vi "TrajAverage.vi"(8 "error in (no error)":errorcluster, 11 "ForceField in":refnum<class "ForceField.lvclass">) -> (0 "error out":errorcluster, 3 "ForceField out":refnum<class "ForceField.lvclass">)   [LabVIEW 2014, in "ForceField.lvclass"]
uses:
  ForceField.lvclass
  TypeDef/AnkleTrajPt.ctl
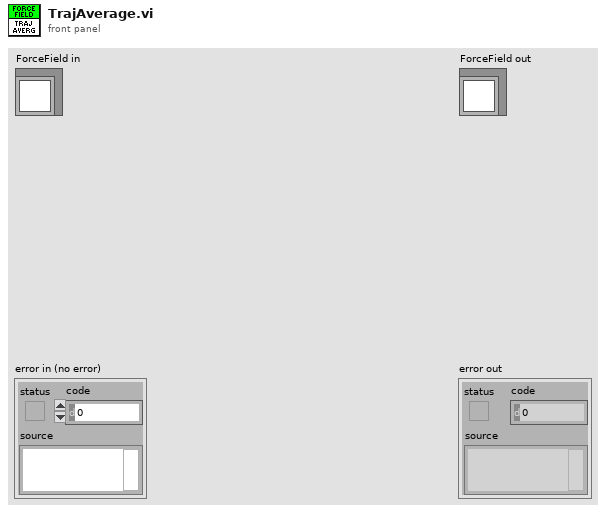
[diagram p1: front panel]
types:
  T1 = typedef "ForceField.lvclass/AnkleTrajPt.ctl" = cluster{"P1":dbl[], "P2":dbl[], "P1-P2":dbl[], "(P1-P2)^2":dbl}
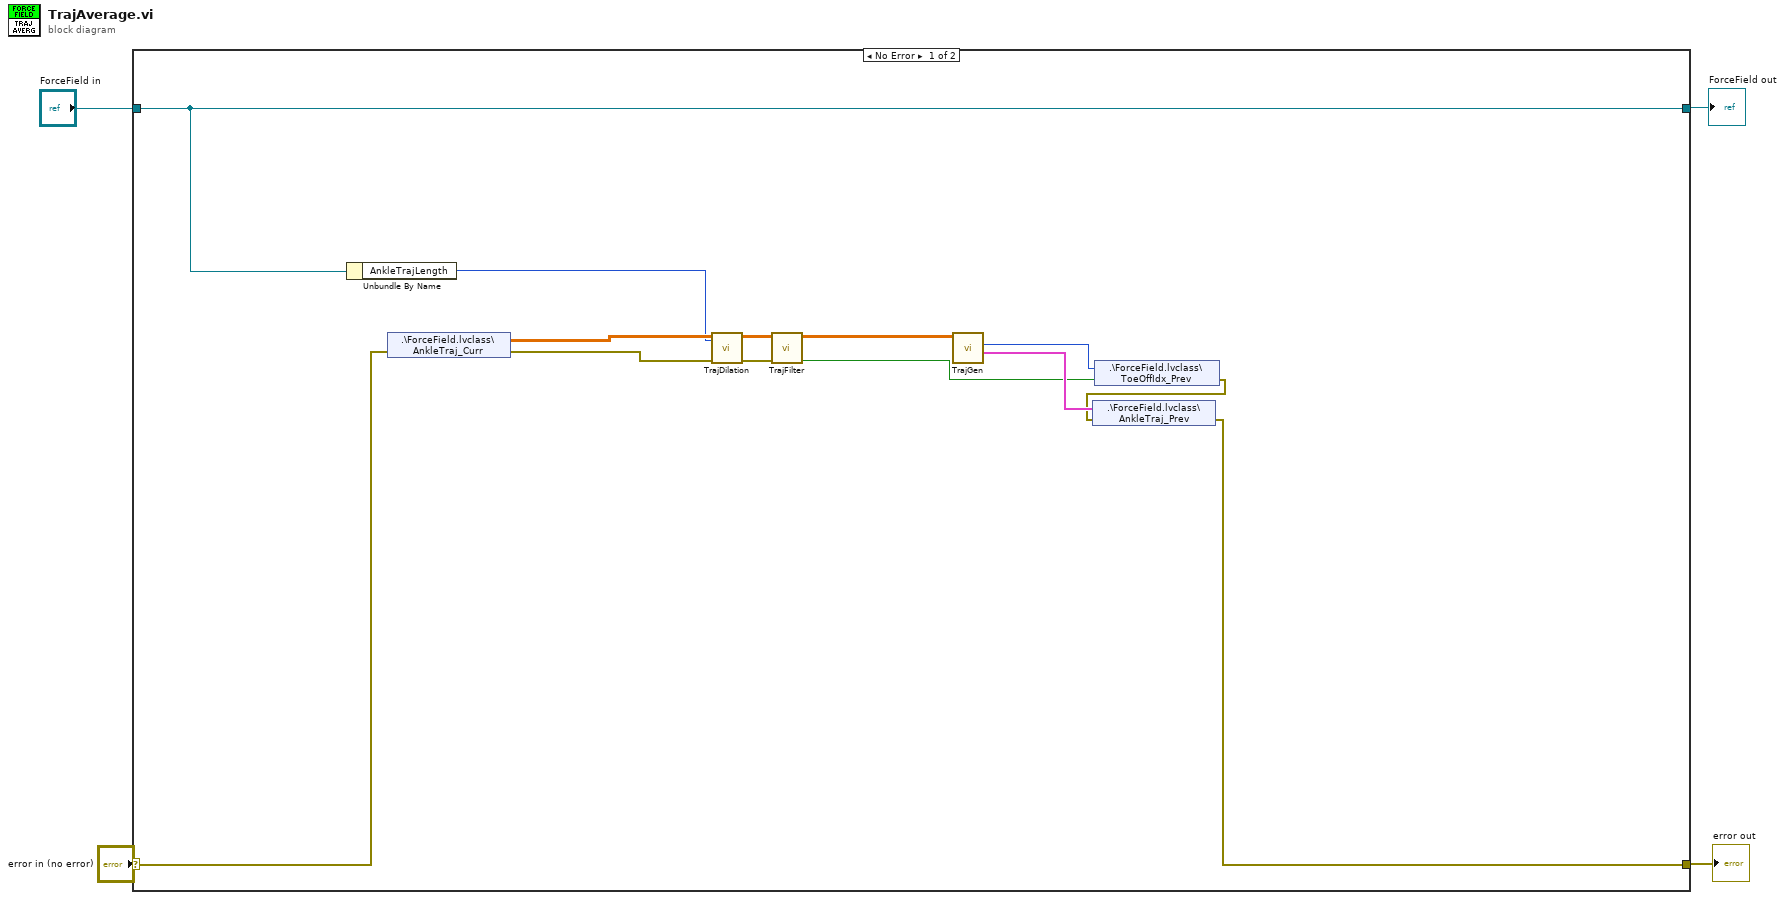
[diagram p0: block diagram]
diagram:
  n1 = case shown="No Error" "error in (no error)" {
    selector: "error in (no error)" -> [w14 w18]
    tunnel: [w7 w18] -> w3
    tunnel: [w13 w17] -> w1
    tunnel: "ForceField in" -> [w13 w17]
    frame No Error {
      n2 = Unbundle By Name(w13) -> ("AnkleTrajLength"=w12:i32)
      n3 = shared-variable ".\\ForceField.lvclass\\AnkleTraj_Curr"(error in=w14) -> (w16:dbl[][], error out=w6:errorcluster)
      n4 = call "TrajDilation.vi"("Length"=w12, "TrajBeforeDilation"=w16) -> ("TrajAfterDilation"=w15:dbl[][])  [unwired: 9 in]
      n5 = call "TrajFilter.vi"("AnkleTraj_Init"=w6, "CurrentTraj"=w15) -> ("AnkleTraj_Init 2"=w5:bool, "AverageTraj"=w11:dbl[][])  [unwired: 6 in]
      n6 = call "TrajGen.vi"("AnkleTraj"=w11) -> ("AnkleTraj"=w10:T1[], "ToeOffIdx"=w9:i32)  [unwired: 5 in, 2 out]
      n7 = shared-variable ".\\ForceField.lvclass\\ToeOffIdx_Prev"(w9, error in=w5) -> (error out=w8:errorcluster)
      n8 = shared-variable ".\\ForceField.lvclass\\AnkleTraj_Prev"(w10, error in=w8) -> (error out=w7:errorcluster)
    }
    frame Error {
    }
  }
  "error out" <- w3
  "ForceField out" <- w1
